vi "Post-Install Custom Action.vi"(10 "variant":variant) -> (0 "error out":errorcluster)   [LabVIEW 2013]
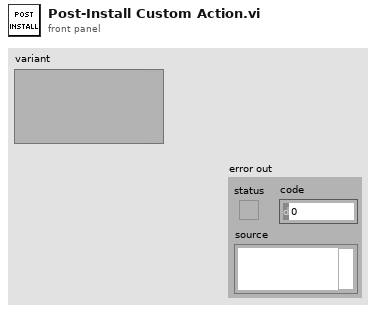
[diagram p1: front panel]
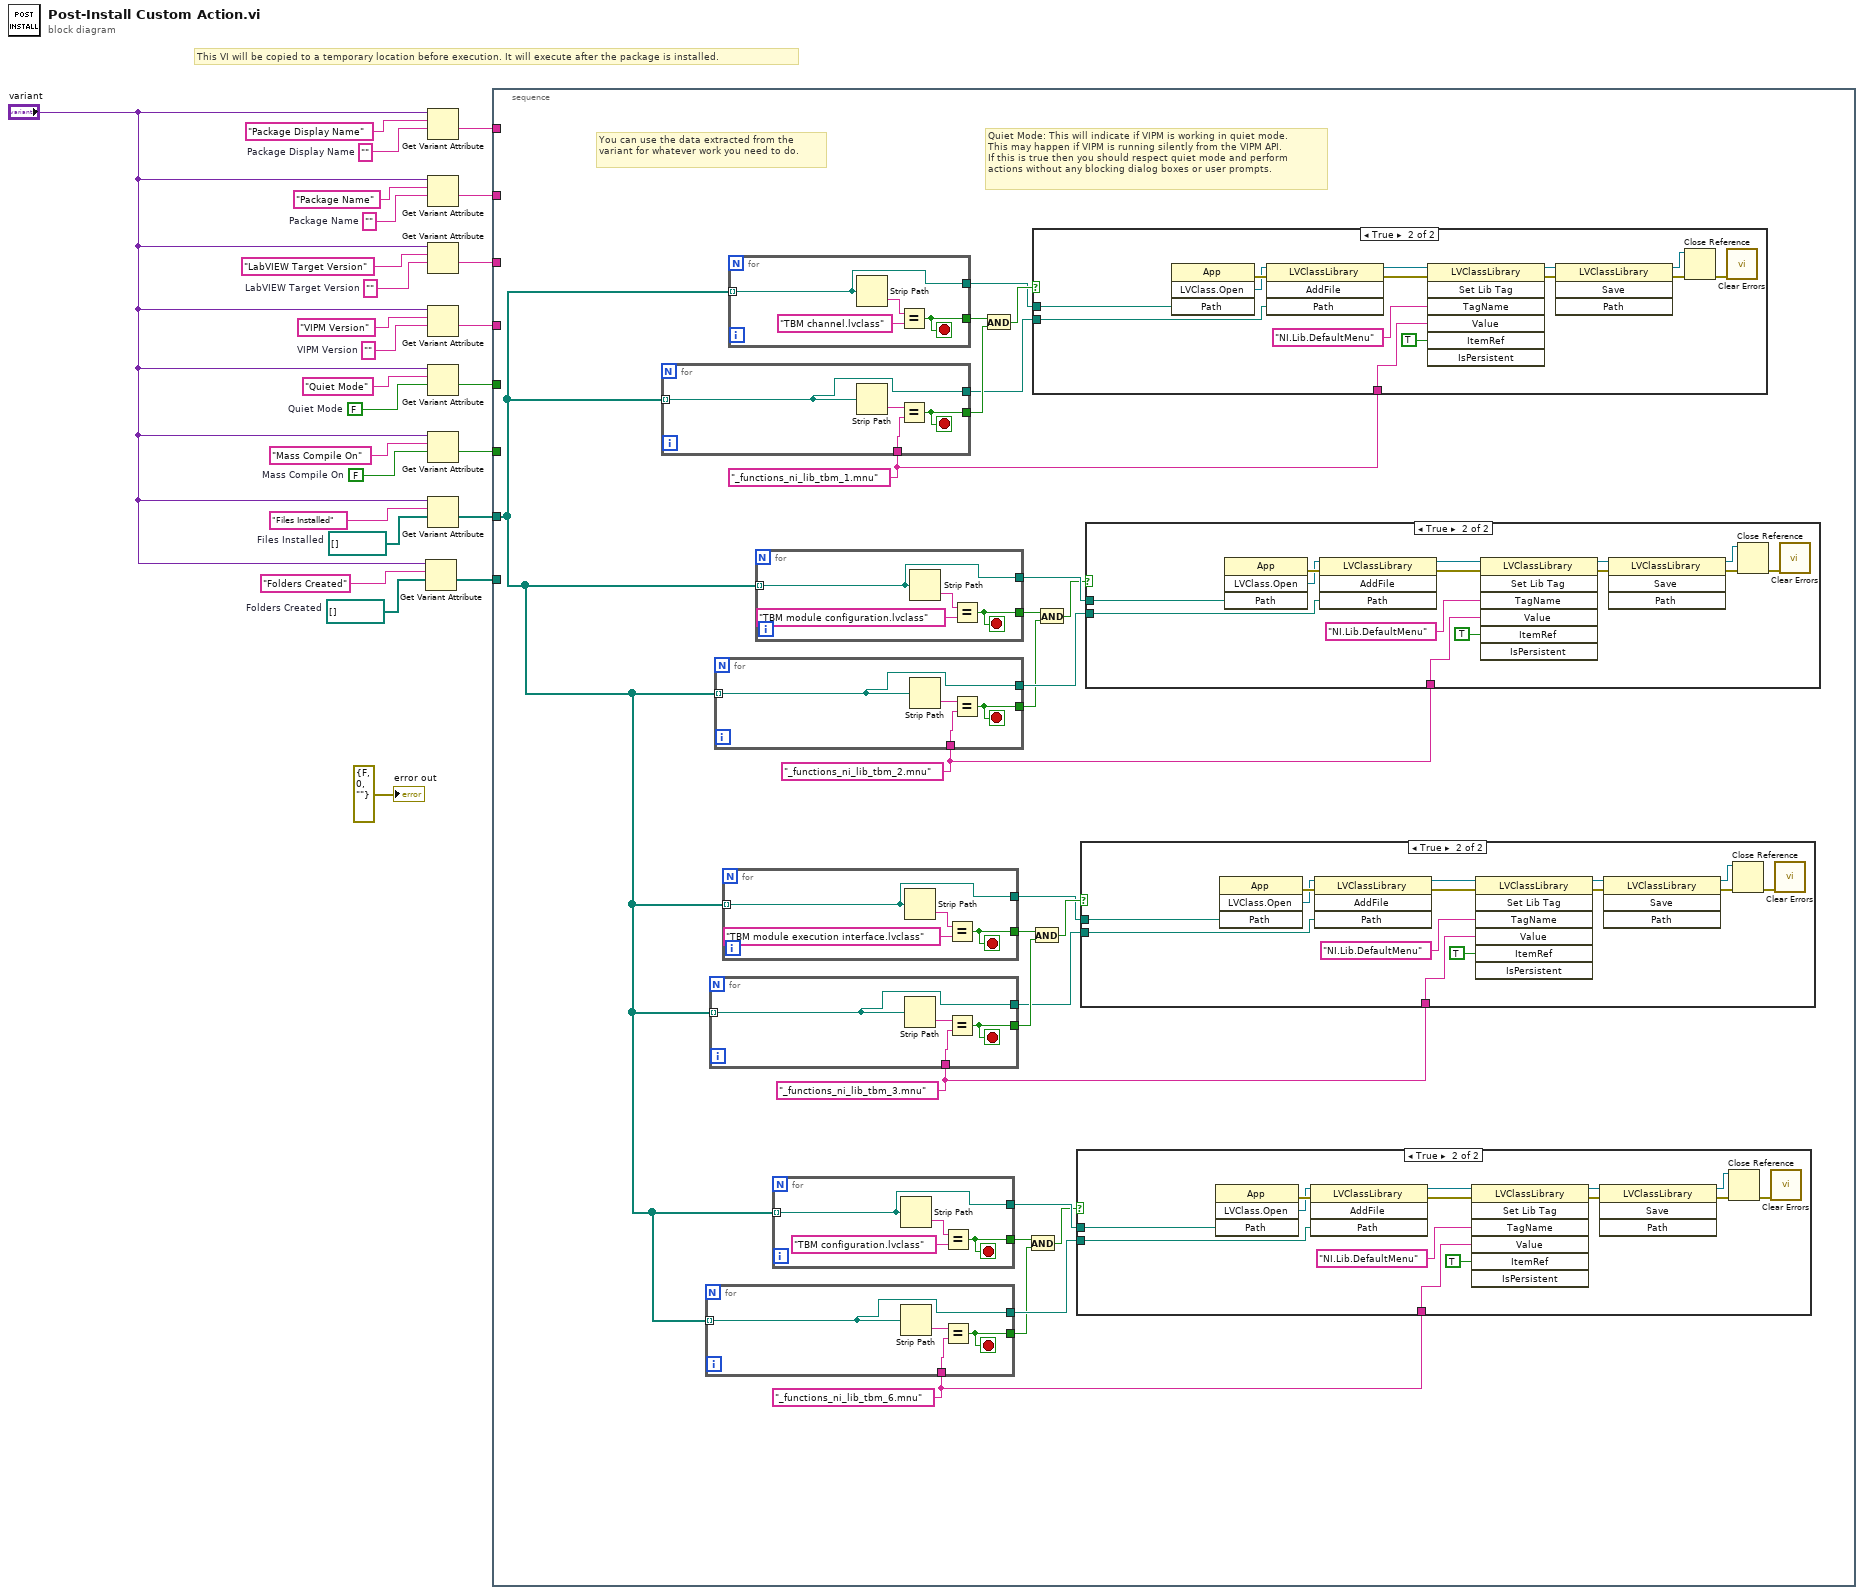
[diagram p0: block diagram]
diagram:
  w1 = path[] []  # Folders Created
  w2 = path[] []  # Files Installed
  w8 = FALSE  # Mass Compile On
  w9 = ""  # Package Display Name
  w16 = FALSE  # Quiet Mode
  w19 = ""  # VIPM Version
  w21 = ""  # LabVIEW Target Version
  w23 = ""  # Package Name
  # "This VI will be copied to a temporary location before execution. It will execute after the package is installed."
  n1 = Get Variant Attribute(Variant="variant", name="Folders Created", default value (empty Variant)=w1) -> (value=w6:path[])  [unwired: 1 in, 3 out]
  n2 = Get Variant Attribute(Variant="variant", name="Package Display Name", default value (empty Variant)=w9) -> (value=w15:string)  [unwired: 1 in, 3 out]
  n3 = Get Variant Attribute(Variant="variant", name="Package Name", default value (empty Variant)=w23) -> (value=w14:string)  [unwired: 1 in, 3 out]
  n4 = Get Variant Attribute(Variant="variant", name="LabVIEW Target Version", default value (empty Variant)=w21) -> (value=w13:string)  [unwired: 1 in, 3 out]
  n5 = Get Variant Attribute(Variant="variant", name="VIPM Version", default value (empty Variant)=w19) -> (value=w12:string)  [unwired: 1 in, 3 out]
  n6 = Get Variant Attribute(Variant="variant", name="Quiet Mode", default value (empty Variant)=w16) -> (value=w11:bool)  [unwired: 1 in, 3 out]
  n7 = Get Variant Attribute(Variant="variant", name="Mass Compile On", default value (empty Variant)=w8) -> (value=w10:bool)  [unwired: 1 in, 3 out]
  n8 = Get Variant Attribute(Variant="variant", name="Files Installed", default value (empty Variant)=w2) -> (value=w5:path[])  [unwired: 1 in, 3 out]
  n9 = stacked-sequence {
    tunnel: w15 -> [_]
    tunnel: w14 -> [_]
    tunnel: w13 -> [_]
    tunnel: w12 -> [_]
    tunnel: w11 -> [_]
    tunnel: w10 -> [_]
    tunnel: w5 -> [w27]
    tunnel: w6 -> [_]
    frame #0 {
      w33 = "_functions_ni_lib_tbm_6.mnu" ("pattern")
      w34 = "_functions_ni_lib_tbm_3.mnu" ("pattern")
      w45 = "_functions_ni_lib_tbm_2.mnu" ("pattern")
      w46 = "_functions_ni_lib_tbm_1.mnu" ("pattern")
      # "Quiet Mode: This will indicate if VIPM is working in quiet mode.\nThis may happen if VIPM is running silently from the VIPM API.\nIf this is true then you should respect quiet mode and perform\nactions without any blocking dialog boxes or user prompts."
      # "You can use the data extracted from the variant for whatever work you need to do."
      n10 = for {
        tunnel: w27 -> [w132] mode=indexing
        tunnel: [w132] -> w47
        tunnel: [w134] -> w51
        tunnel: w46 -> [w133]
        stop <- w134 stop-if-true
        n11 = Strip Path(path=w132) -> (name=w135:string)  [unwired: 1 out]
        n12 = Equal?(x=w135, y=w133) -> (x = y?=w134:bool)
      }
      n13 = for {
        tunnel: w27 -> [w66] mode=indexing
        tunnel: [w66] -> w32
        tunnel: [w68] -> w28
        tunnel: w33 -> [w67]
        stop <- w68 stop-if-true
        n14 = Strip Path(path=w66) -> (name=w69:string)  [unwired: 1 out]
        n15 = Equal?(x=w69, y=w67) -> (x = y?=w68:bool)
      }
      n16 = for {
        tunnel: w27 -> [w88] mode=indexing
        tunnel: [w88] -> w35
        tunnel: [w90] -> w39
        tunnel: w34 -> [w89]
        stop <- w90 stop-if-true
        n17 = Strip Path(path=w88) -> (name=w91:string)  [unwired: 1 out]
        n18 = Equal?(x=w91, y=w89) -> (x = y?=w90:bool)
      }
      n19 = for {
        tunnel: w27 -> [w110] mode=indexing
        tunnel: [w110] -> w44
        tunnel: [w112] -> w40
        tunnel: w45 -> [w111]
        stop <- w112 stop-if-true
        n20 = Strip Path(path=w110) -> (name=w113:string)  [unwired: 1 out]
        n21 = Equal?(x=w113, y=w111) -> (x = y?=w112:bool)
      }
      n22 = for {
        tunnel: w27 -> [w92] mode=indexing
        tunnel: [w92] -> w36
        tunnel: [w93] -> w38
        stop <- w93 stop-if-true
        n23 = Strip Path(path=w92) -> (name=w94:string)  [unwired: 1 out]
        n24 = Equal?(x=w94, y="TBM module execution interface.lvclass" ("pattern")) -> (x = y?=w93:bool)
      }
      n25 = for {
        tunnel: w27 -> [w136] mode=indexing
        tunnel: [w136] -> w48
        tunnel: [w137] -> w50
        stop <- w137 stop-if-true
        n26 = Strip Path(path=w136) -> (name=w138:string)  [unwired: 1 out]
        n27 = Equal?(x=w138, y="TBM channel.lvclass" ("pattern")) -> (x = y?=w137:bool)
      }
      n28 = for {
        tunnel: w27 -> [w114] mode=indexing
        tunnel: [w114] -> w43
        tunnel: [w115] -> w41
        stop <- w115 stop-if-true
        n29 = Strip Path(path=w114) -> (name=w116:string)  [unwired: 1 out]
        n30 = Equal?(x=w116, y="TBM module configuration.lvclass" ("pattern")) -> (x = y?=w115:bool)
      }
      n31 = for {
        tunnel: w27 -> [w70] mode=indexing
        tunnel: [w70] -> w31
        tunnel: [w71] -> w29
        stop <- w71 stop-if-true
        n32 = Strip Path(path=w70) -> (name=w72:string)  [unwired: 1 out]
        n33 = Equal?(x=w72, y="TBM configuration.lvclass" ("pattern")) -> (x = y?=w71:bool)
      }
      n34 = And(x=w50, y=w51) -> (x .and. y?=w49:bool)
      n35 = And(x=w29, y=w28) -> (x .and. y?=w30:bool)
      n36 = And(x=w38, y=w39) -> (x .and. y?=w37:bool)
      n37 = case shown="True" w49 {
        tunnel: w48 -> [_ w120]
        tunnel: w47 -> [_ w119]
        tunnel: w46 -> [_ w118]
        frame False {
        }
        frame True {
          n38 = invoke class="App" method="LVClass.Open"("Path"=w120) -> (error out=w131:errorcluster, "LVClass.Open"=w128:refnum<vi>)  [unwired: 3 in, 2 out]
          n39 = invoke class="LVClassLibrary" method="AddFile"(reference=w128, error in=w131, "Path"=w119) -> (reference out=w127:refnum<vi>, error out=w129:errorcluster)  [unwired: 1 in, 2 out]
          n40 = invoke class="LVClassLibrary" method="Set Lib Tag"(reference=w127, error in=w129, "TagName"="NI.Lib.DefaultMenu" ("Tag Name"), "Value"=w118, "ItemRef"=TRUE ("Is Persistent")) -> (reference out=w123:refnum<vi>, error out=w126:errorcluster)  [unwired: 2 in, 5 out]
          n41 = invoke class="LVClassLibrary" method="Save"(reference=w123, error in=w126) -> (reference out=w122:refnum<vi>, error out=w124:errorcluster)  [unwired: 2 in, 2 out]
          n42 = Close Reference(reference=w122, error in (no error)=w124) -> (error out=w130:errorcluster)
          n43 = call <vilib>:"Clear Errors.vi"("error in (no error)"=w130) -> ()  [unwired: 6 in, 1 out]
        }
      }
      n44 = And(x=w41, y=w40) -> (x .and. y?=w42:bool)
      n45 = case shown="True" w30 {
        tunnel: w31 -> [_ w54]
        tunnel: w32 -> [_ w53]
        tunnel: w33 -> [_ w52]
        frame False {
        }
        frame True {
          n46 = invoke class="App" method="LVClass.Open"("Path"=w54) -> (error out=w65:errorcluster, "LVClass.Open"=w62:refnum<vi>)  [unwired: 3 in, 2 out]
          n47 = invoke class="LVClassLibrary" method="AddFile"(reference=w62, error in=w65, "Path"=w53) -> (reference out=w61:refnum<vi>, error out=w63:errorcluster)  [unwired: 1 in, 2 out]
          n48 = invoke class="LVClassLibrary" method="Set Lib Tag"(reference=w61, error in=w63, "TagName"="NI.Lib.DefaultMenu" ("Tag Name"), "Value"=w52, "ItemRef"=TRUE ("Is Persistent")) -> (reference out=w57:refnum<vi>, error out=w60:errorcluster)  [unwired: 2 in, 5 out]
          n49 = invoke class="LVClassLibrary" method="Save"(reference=w57, error in=w60) -> (reference out=w56:refnum<vi>, error out=w58:errorcluster)  [unwired: 2 in, 2 out]
          n50 = Close Reference(reference=w56, error in (no error)=w58) -> (error out=w64:errorcluster)
          n51 = call <vilib>:"Clear Errors.vi"("error in (no error)"=w64) -> ()  [unwired: 6 in, 1 out]
        }
      }
      n52 = case shown="True" w37 {
        tunnel: w36 -> [_ w76]
        tunnel: w35 -> [_ w75]
        tunnel: w34 -> [_ w74]
        frame False {
        }
        frame True {
          n53 = invoke class="App" method="LVClass.Open"("Path"=w76) -> (error out=w87:errorcluster, "LVClass.Open"=w84:refnum<vi>)  [unwired: 3 in, 2 out]
          n54 = invoke class="LVClassLibrary" method="AddFile"(reference=w84, error in=w87, "Path"=w75) -> (reference out=w83:refnum<vi>, error out=w85:errorcluster)  [unwired: 1 in, 2 out]
          n55 = invoke class="LVClassLibrary" method="Set Lib Tag"(reference=w83, error in=w85, "TagName"="NI.Lib.DefaultMenu" ("Tag Name"), "Value"=w74, "ItemRef"=TRUE ("Is Persistent")) -> (reference out=w79:refnum<vi>, error out=w82:errorcluster)  [unwired: 2 in, 5 out]
          n56 = invoke class="LVClassLibrary" method="Save"(reference=w79, error in=w82) -> (reference out=w78:refnum<vi>, error out=w80:errorcluster)  [unwired: 2 in, 2 out]
          n57 = Close Reference(reference=w78, error in (no error)=w80) -> (error out=w86:errorcluster)
          n58 = call <vilib>:"Clear Errors.vi"("error in (no error)"=w86) -> ()  [unwired: 6 in, 1 out]
        }
      }
      n59 = case shown="True" w42 {
        tunnel: w43 -> [_ w98]
        tunnel: w44 -> [_ w97]
        tunnel: w45 -> [_ w96]
        frame False {
        }
        frame True {
          n60 = invoke class="App" method="LVClass.Open"("Path"=w98) -> (error out=w109:errorcluster, "LVClass.Open"=w106:refnum<vi>)  [unwired: 3 in, 2 out]
          n61 = invoke class="LVClassLibrary" method="AddFile"(reference=w106, error in=w109, "Path"=w97) -> (reference out=w105:refnum<vi>, error out=w107:errorcluster)  [unwired: 1 in, 2 out]
          n62 = invoke class="LVClassLibrary" method="Set Lib Tag"(reference=w105, error in=w107, "TagName"="NI.Lib.DefaultMenu" ("Tag Name"), "Value"=w96, "ItemRef"=TRUE ("Is Persistent")) -> (reference out=w101:refnum<vi>, error out=w104:errorcluster)  [unwired: 2 in, 5 out]
          n63 = invoke class="LVClassLibrary" method="Save"(reference=w101, error in=w104) -> (reference out=w100:refnum<vi>, error out=w102:errorcluster)  [unwired: 2 in, 2 out]
          n64 = Close Reference(reference=w100, error in (no error)=w102) -> (error out=w108:errorcluster)
          n65 = call <vilib>:"Clear Errors.vi"("error in (no error)"=w108) -> ()  [unwired: 6 in, 1 out]
        }
      }
    }
  }
  "error out" <- errorcluster {"status"=FALSE, "code"=0, "source"=""} ("error out")
